vi "FRCts20_Backend_GenTeamList.vi"(8 "error in (no error)":errorcluster, 11 "Competitions":T1) -> (0 "error out":errorcluster, 2 "TeamList_Flattened":string, 3 "Competitions Oot":T1)   [LabVIEW 2014, in "FRCts20_Backend_Engine_Deprecated.lvlib"]
uses:
  FRCts20_Backend_Engine_Deprecated.lvlib
  FRCts20_Backend_TeamDataDfn.ctl
  FRCts20_Backend_Controls.lvlib
  FRCts20_Backend_TeamDfn.ctl
  FRCts20_Backend_IssueDfn.ctl
  FRCts20_Backend_TeamList.ctl
  FRCts20_Backend_Team_Info.ctl
  FRCts20_Backend_Note.ctl
  FRCts20_Backend_Note_list.ctl
  FRCts20_Backend_request_info.ctl
  FRCts20_Backend_IssueTeamList.ctl
  FRCts20_Backend_Competition_Info.ctl
  FRCts20_Backend_Division_Info.ctl
  FRCts20_Backend_Division.ctl
  FRCts20_Backend_Division_List.ctl
  FRCts20_Backend_Competition.ctl
  FRCts20_Backend_Competition_List.ctl
panel:
  in  "TeamList_Ref":T15
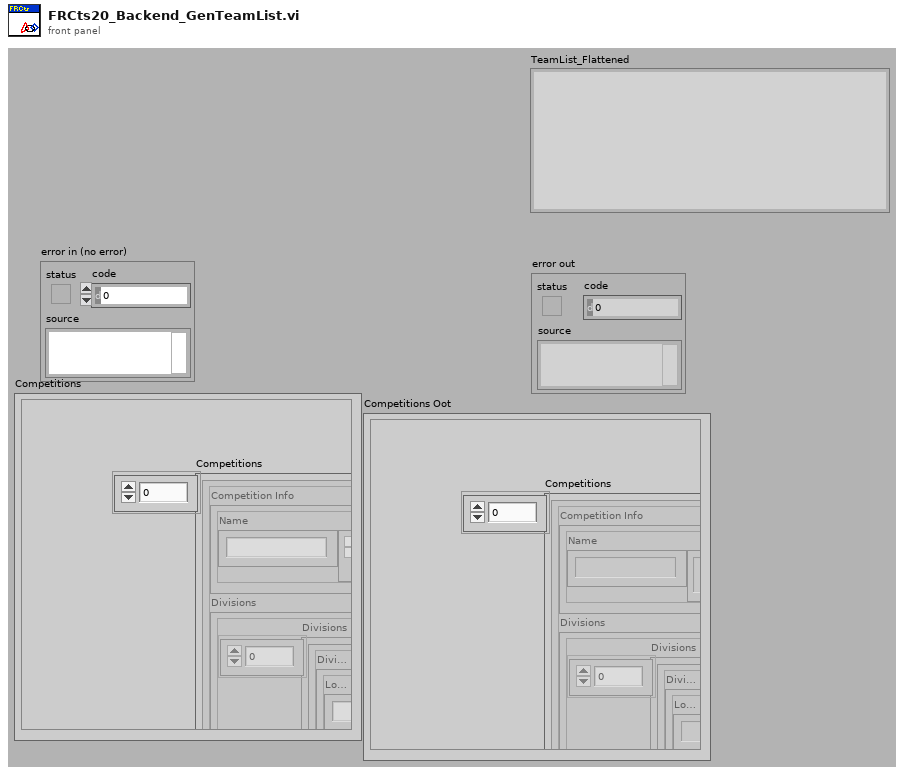
[diagram p1: front panel]
types:
  T1 = typedef "FRCts20_Backend_Controls.lvlib/FRCts20_Backend_Competition_List.ctl" = cluster{"Competitions":T2[]}
  T2 = typedef "FRCts20_Backend_Controls.lvlib/FRCts20_Backend_Competition.ctl" = cluster{"Competition Info":T3, "Divisions":T4}
  T3 = typedef "FRCts20_Backend_Controls.lvlib/FRCts20_Backend_Competition_Info.ctl" = cluster{"Name":string, "Start Date":timestamp, "Duration":u8}
  T4 = typedef "FRCts20_Backend_Controls.lvlib/FRCts20_Backend_Division_List.ctl" = cluster{"Divisions":T5[]}
  T5 = typedef "FRCts20_Backend_Controls.lvlib/FRCts20_Backend_Division.ctl" = cluster{"Division Info":T6, "TeamData":T7}
  T6 = typedef "FRCts20_Backend_Controls.lvlib/FRCts20_Backend_Division_Info.ctl" = cluster{"Location":string}
  T7 = typedef "FRCts20_Backend_Controls.lvlib/FRCts20_Backend_TeamDataDfn.ctl" = cluster{"Team":T8[]}
  T8 = typedef "FRCts20_Backend_Controls.lvlib/FRCts20_Backend_TeamDfn.ctl" = cluster{"Team Info":T9, "IssueList":T10}
  T9 = typedef "FRCts20_Backend_Controls.lvlib/FRCts20_Backend_Team_Info.ctl" = cluster{"TeamNumber":u16, "SWType":string}
  T10 = typedef "FRCts20_Backend_Controls.lvlib/FRCts20_Backend_IssueTeamList.ctl" = cluster{"Issues":T11[]}
  T11 = typedef "FRCts20_Backend_Controls.lvlib/FRCts20_Backend_IssueDfn.ctl" = cluster{"Notes":T12, "Info":T14}
  T12 = typedef "FRCts20_Backend_Controls.lvlib/FRCts20_Backend_Note_list.ctl" = cluster{"Notes":T13[]}
  T13 = typedef "FRCts20_Backend_Controls.lvlib/FRCts20_Backend_Note.ctl" = cluster{"Time Entered":timestamp, "Author":string, "Text":string}
  T14 = typedef "FRCts20_Backend_Controls.lvlib/FRCts20_Backend_request_info.ctl" = cluster{"Status":enum16{"Open", "In Work", "Closed"}, "Open Date":timestamp, "Description":string, "Last Update":timestamp, "Closed Date":timestamp, "Solution Index":i32}
  T15 = typedef "FRCts20_Backend_Controls.lvlib/FRCts20_Backend_TeamList.ctl" = cluster{"Team":cluster{"TeamNumber":u16, "Location":string}[]}
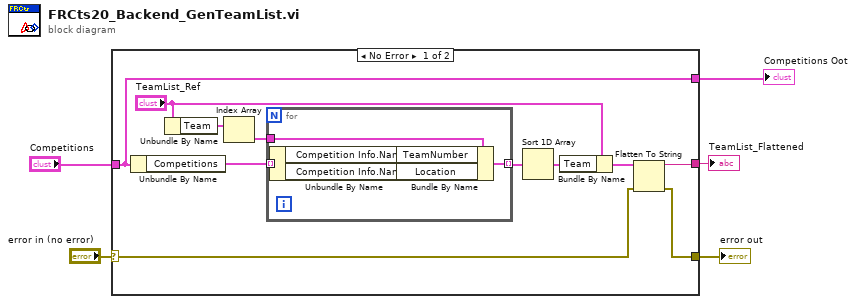
[diagram p0: block diagram]
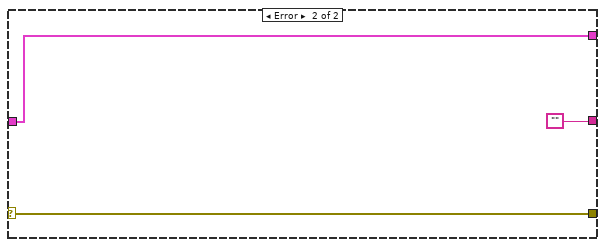
[diagram p2: hidden frame]
diagram:
  n1 = case shown="No Error" "error in (no error)" {
    selector: "error in (no error)" -> [w7 w24]
    tunnel: [w6 w24] -> w4
    tunnel: "Competitions" -> [w10 w22]
    tunnel: [w10 w22] -> w2
    tunnel: [w8 ""] -> w3
    frame No Error {
      n2 = Unbundle By Name(w10) -> ("Competitions"=w16:T2[])
      n3 = Unbundle By Name("TeamList_Ref") -> ("Team"=w15:cluster{"TeamNumber":u16, "Location":string}[])
      n4 = Index Array(array=w15) -> (element=w14:cluster{"TeamNumber":u16, "Location":string})  [unwired: 1 in]
      n5 = for {
        tunnel: w16 -> [w21] mode=indexing
        tunnel: w14 -> [w20]
        tunnel: [w17] -> w12 mode=indexing
        n6 = Unbundle By Name(w21) -> ("Competition Info.Name"=w19:string, "Competition Info.Name"=w18:string)
        n7 = Bundle By Name(cluster=w20, "TeamNumber"=w19, "Location"=w18) -> (w17:cluster{"TeamNumber":u16, "Location":string})
      }
      n8 = Sort 1D Array(array=w12) -> (sorted array=w11:cluster{"TeamNumber":u16, "Location":string}[])
      n9 = Bundle By Name(cluster="TeamList_Ref", "Team"=w11) -> (w9:T15)
      n10 = Flatten To String(anything=w9, error in (no error)=w7) -> (data string=w8:string, error out=w6:errorcluster)  [unwired: 2 in, 1 out]
    }
    frame Error {
    }
  }
  "error out" <- w4
  "TeamList_Flattened" <- w3
  "Competitions Oot" <- w2
